vi "code (realtime).vi"() -> ()   [LabVIEW 2009]
uses:
  <vilib>/userDefined/High Color/IMAQdx.ctl
  <vilib>/Utility/file.llb/Write To Spreadsheet File (DBL).vi
  <vilib>/vision/driver/NI_Vision_Acquisition_Software.lvlib
panel:
  in  "START":bool
  in  "AVI FILE":path
  out "x/y":dbl
  in  "file path to save data":path
  out "Array":dbl[][](array[numeric])
  out "time":i32
  in  "SET":bool
  in  "CODE":bool
  in  "stop":bool
  in  "PG":bool
  in  "SG":bool
  in  "SF":bool
  in  "C":bool
  in  "PF":bool
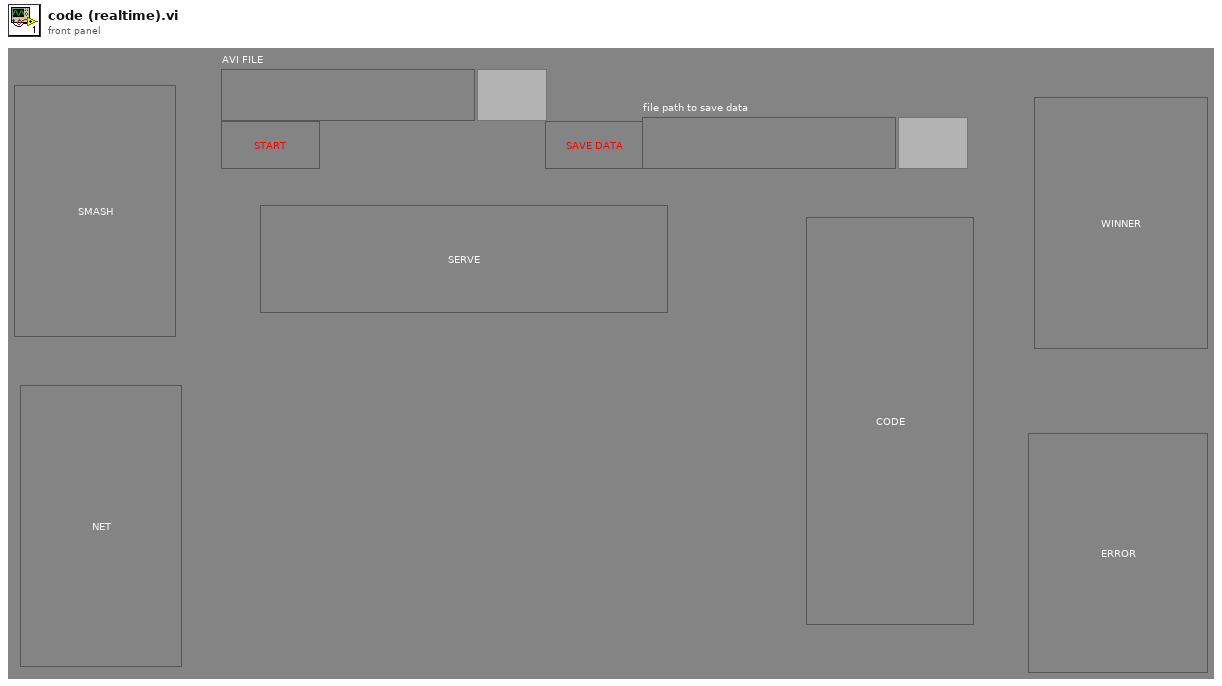
[diagram p1: front panel]
types:
  T1 = typedef "IMAQdx.ctl" = refnum<k21>
  T2 = typedef "AviRefnum.ctl" = refnum<k1>
  T3 = typedef "IMAQ Image.ctl" = refnum<image>
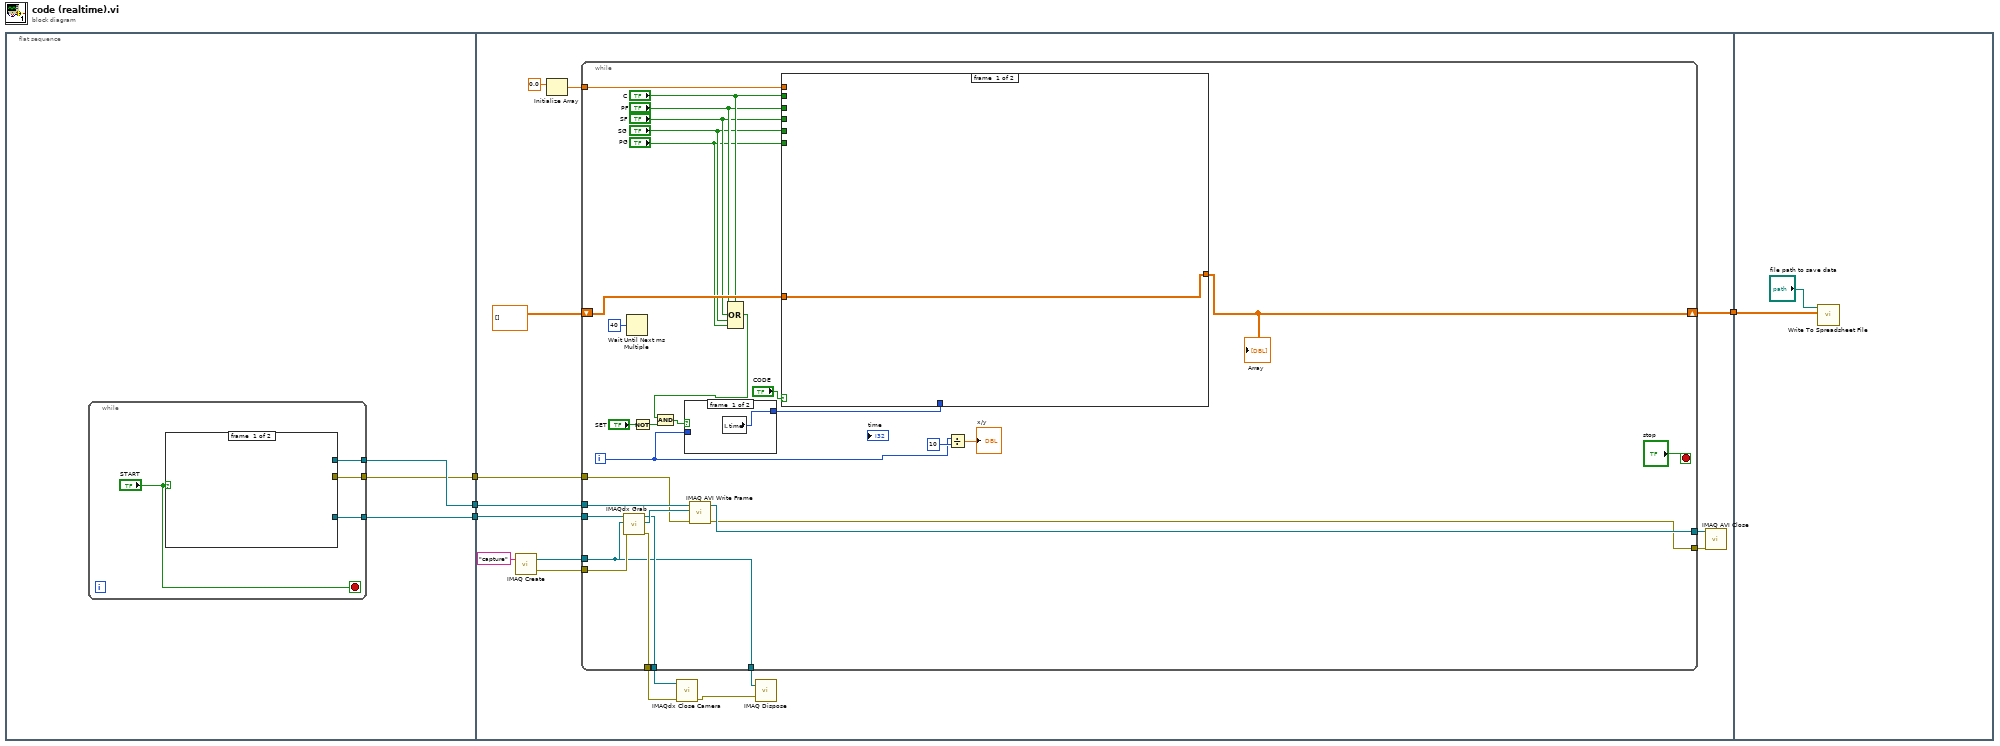
[diagram p0: block diagram]
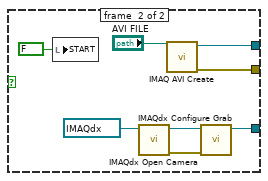
[diagram p2: hidden frame]
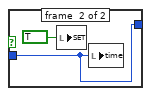
[diagram p3: hidden frame]
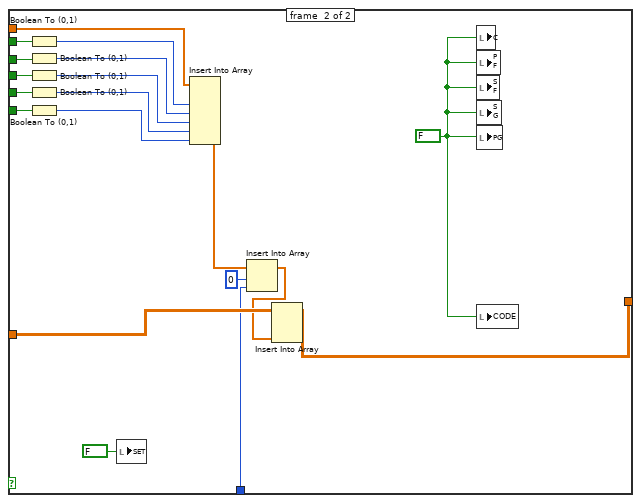
[diagram p4: hidden frame]
diagram:
  n1 = flat-sequence {
    tunnel: [w7] -> w3
    tunnel: [w6] -> w2
    tunnel: [w5] -> w1
    tunnel: [w32] -> w4
    tunnel: w3 -> [w29]
    tunnel: w2 -> [w27]
    tunnel: w1 -> [w26]
    tunnel: w4 -> [w89]
    frame #0 {
      n2 = while {
        tunnel: [w11] -> w7
        tunnel: [w10] -> w6
        tunnel: [w9] -> w5
        stop <- "START" stop-if-true
        n3 = case shown="True" "START" {
          tunnel: [_ w16] -> w11
          tunnel: [_ w14] -> w10
          tunnel: [_ w13] -> w9
          frame #0 {
          }
          frame #1 {
            n4 = local write "START"(FALSE ("START")) -> ()
            n5 = call <vilib>:"IMAQdx Open Camera.vi"("Session In"=T1 "cam1") -> ("error out"=w18:errorcluster, "Session Out"=w17:T1)  [unwired: 9 in]
            n6 = call "IMAQ AVI Create"("AVI Path"="AVI FILE") -> ("error out"=w13:errorcluster, "Avi Refnum"=w14:T2)  [unwired: 9 in]
            n7 = call <vilib>:"IMAQdx Configure Grab.vi"("error in"=w18, "Session In"=w17) -> ("Session Out"=w16:T1)  [unwired: 8 in, 1 out]
          }
        }
      }
    }
    frame #1 {
      n8 = call "IMAQ Create"("Image Name"="capture") -> ("New Image"=w30:T3, "error out"=w28:errorcluster)  [unwired: 4 in]
      n9 = Initialize Array(0.0 ("element")) -> (w34:dbl[])  [unwired: 1 in]
      n10 = while {
        tunnel: w34 -> [w61]
        shift-right: [w62] -> w32
        shift-left: dbl[][] [] ("Array") -> [w60]
        tunnel: w30 -> [w36]
        tunnel: w29 -> [w45]
        tunnel: w28 -> [w44]
        tunnel: w27 -> [w42]
        tunnel: w26 -> [w41]
        tunnel: [w40] -> w25
        tunnel: [w39] -> w24
        tunnel: [w38] -> w23
        tunnel: [w37] -> w22
        tunnel: [w36] -> w20
        i -> [w56]
        stop <- "stop" stop-if-true
        n11 = call <vilib>:"IMAQdx Grab.vi"("error in"=w44, "Image In"=w36, "Session In"=w45) -> ("error out"=w37:errorcluster, "Image Out"=w43:T3, "Session Out"=w38:T1)  [unwired: 5 in, 1 out]
        n12 = Wait Until Next ms Multiple(millisecond multiple=u32 40) -> ()  [unwired: 1 out]
        n13 = Not(x="SET") -> (.not. x?=w47:bool)
        n14 = call "IMAQ AVI Write Frame"("error in (no error)"=w41, "Image"=w43, "Avi Refnum"=w42) -> ("error out"=w39:errorcluster, "Avi Refnum (duplicate)"=w40:T2)  [unwired: 7 in]
        n15 = Compound Arithmetic op=OR("C", "PF", "SF", "SG", "PG") -> (w49:bool)
        n16 = And(x=w49, y=w47) -> (x .and. y?=w48:bool)
        n17 = case shown="True" w48 {
          tunnel: w56 -> [_ w67]
          tunnel: [w65 w67] -> w58
          frame #0 {
            n18 = local read "time"() -> (w65:i32)
          }
          frame #1 {
            n19 = local write "SET"(TRUE ("SET")) -> ()
            n20 = local write "time"(w67) -> ()
          }
        }
        n21 = case shown="True" "CODE" {
          tunnel: "PG" -> [_ w83]
          tunnel: "SG" -> [_ w87]
          tunnel: "SF" -> [_ w86]
          tunnel: "PF" -> [_ w85]
          tunnel: "C" -> [_ w84]
          tunnel: [w68 w75] -> w62
          tunnel: w61 -> [_ w77]
          tunnel: w60 -> [w68 w76]
          tunnel: w58 -> [_ w73]
          frame #0 {
          }
          frame #1 {
            w70 = FALSE ("PG")
            n22 = Boolean To (0,1)(Boolean=w84) -> (0, 1=w82:i16)
            n23 = Boolean To (0,1)(Boolean=w85) -> (0, 1=w81:i16)
            n24 = Boolean To (0,1)(Boolean=w86) -> (0, 1=w80:i16)
            n25 = Boolean To (0,1)(Boolean=w87) -> (0, 1=w79:i16)
            n26 = Boolean To (0,1)(Boolean=w83) -> (0, 1=w78:i16)
            n27 = local write "SET"(FALSE ("SET")) -> ()
            n28 = Insert Into Array(array=w77, new element #1=w82, new element #2=w81, new element #3=w80, new element #4=w79, new element #5=w78) -> (w74:dbl[])  [unwired: 1 in]
            n29 = Insert Into Array(array=w74, index=0, new element=w73) -> (w71:dbl[])
            n30 = Insert Into Array(array=w76, new element=w71) -> (w75:dbl[][])  [unwired: 2 in]
            n31 = local write "C"(w70) -> ()
            n32 = local write "PF"(w70) -> ()
            n33 = local write "SF"(w70) -> ()
            n34 = local write "SG"(w70) -> ()
            n35 = local write "PG"(w70) -> ()
            n36 = local write "CODE"(w70) -> ()
          }
        }
        "Array" <- w62
        n37 = Divide(x=w56, y=10) -> (x/y=→"x/y":dbl)
      }
      n38 = call <vilib>:"IMAQdx Close Camera.vi"("error in"=w22, "Session In"=w23) -> ("error out"=w21:errorcluster)  [unwired: 9 in]
      n39 = call "IMAQ Dispose"("Image"=w20, "error in (no error)"=w21) -> ()  [unwired: 4 in, 1 out]
      n40 = call "IMAQ AVI Close"("error in (no error)"=w24, "Avi Refnum"=w25) -> ()  [unwired: 9 in, 1 out]
    }
    frame #2 {
      n41 = call-poly <vilib>:"Write To Spreadsheet File.vi"("2D data"=w89, "file path (dialog if empty)"="file path to save data") -> ()  [unwired: 6 in, 1 out]
    }
  }
